vi "Gas HHV Initialize.vi"(6 "Manual HHV Mode?":bool, 8 "error in (no error)":errorcluster, 9 "Remote Port":u16, 10 "Propane IP Address":string, 11 "Natural Gas  IP Address":string) -> (0 "error out":errorcluster, 2 "TCP master instance":refnum<class "Modbus Master.lvclass">, 3 "Modbus Master out":refnum<class "Modbus Master.lvclass">)   [LabVIEW 2020]
uses:
  <vilib>/NI/Modbus Library/API/Master/Modbus Master.lvclass
  <vilib>/NI/Modbus Library/API/Wrapper/Create TCP Master.vi
  <vilib>/NI/Modbus Library/API/Wrapper/API Main.lvlib
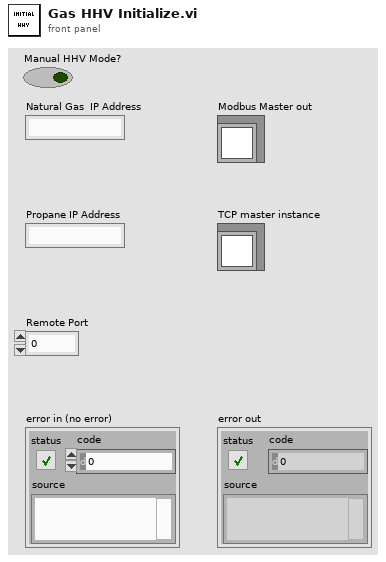
[diagram p1: front panel]
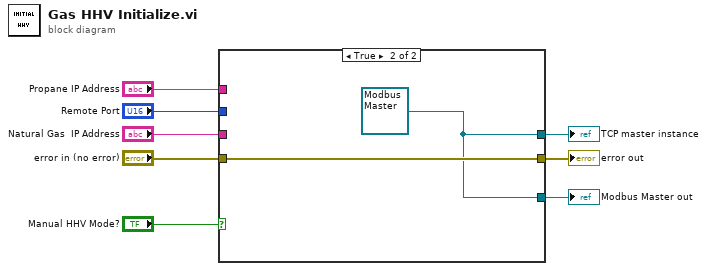
[diagram p0: block diagram]
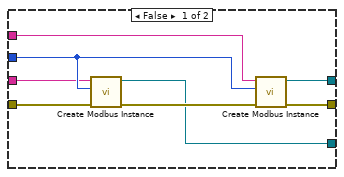
[diagram p2: hidden frame]
diagram:
  n1 = case shown="True" "Manual HHV Mode?" {
    tunnel: [w16 w17] -> w8
    tunnel: "Remote Port" -> [w15 _]
    tunnel: "Propane IP Address" -> [w14 _]
    tunnel: [w13 w18] -> w5
    tunnel: [w11 w17] -> w4
    tunnel: "Natural Gas  IP Address" -> [w10 _]
    tunnel: "error in (no error)" -> [w9 w18]
    frame False {
      n2 = call-poly <vilib>:"Create Modbus Instance.vi"("error in"=w9, "port (502)"=w15, "address"=w10) -> ("error out"=w12:errorcluster, "TCP master instance"=w11:refnum<class "Modbus Master.lvclass">)  [unwired: 7 in]
      n3 = call-poly <vilib>:"Create Modbus Instance.vi"("error in"=w12, "port (502)"=w15, "address"=w14) -> ("error out"=w13:errorcluster, "TCP master instance"=w16:refnum<class "Modbus Master.lvclass">)  [unwired: 7 in]
    }
    frame True {
      w17 = refnum<class "Modbus Master.lvclass"> refnum ("TCP master instance")
    }
  }
  "TCP master instance" <- w8
  "error out" <- w5
  "Modbus Master out" <- w4
